vi "connect.vi"(3 "Connect":bool, 7 "LabVIEW Web Service Request":refnum<class "Web Request.lvclass">) -> ()   [LabVIEW 2014]
uses:
  <vilib>/wsapi/Web Request.lvclass
  controls/UI DataSam.ctl
panel:
  # "Use the Web Service Request input terminal to call the VIs on the Web Services palette. Do not remove it from the connector pane unless you don't need access to the palette."
  # "Each additional control wired to the connector pane will be available as an input in the URL. To include an indicator in terminal-mode output (the default setting), it must also be wired to the connector pane."
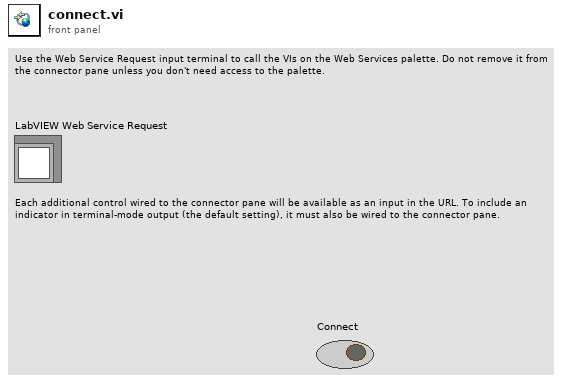
[diagram p1: front panel]
types:
  T1 = typedef "UI DataSam.ctl" = cluster{"Message":string, "Data":variant}
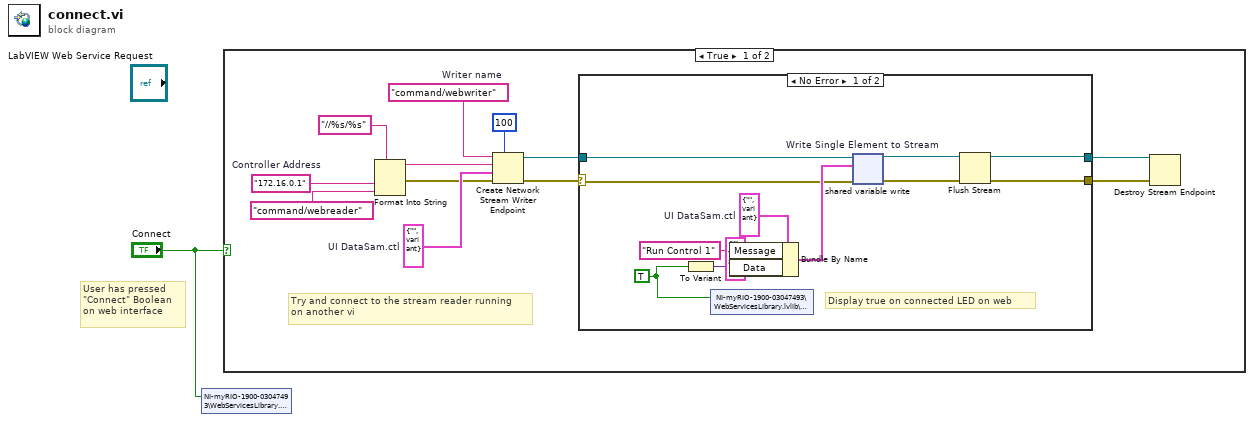
[diagram p0: block diagram]
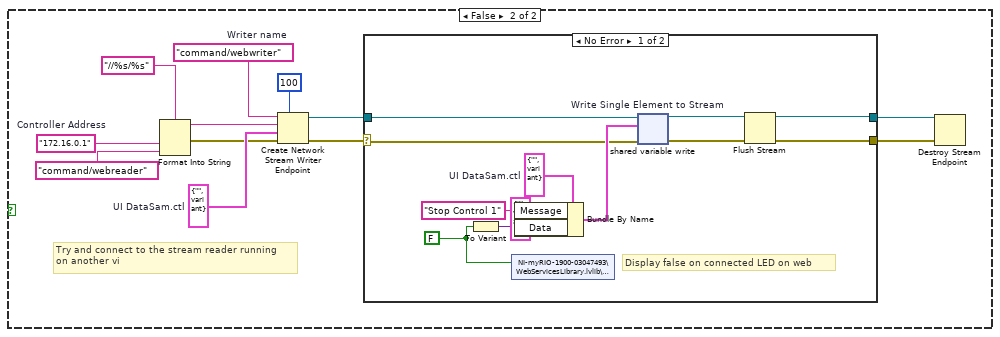
[diagram p3: hidden frame]
diagram:
  # "User has pressed\n\"Connect\" Boolean\non web interface"
  n1 = shared-variable "NI-myRIO-1900-03047493\\WebServicesLibrary.lvlib\\Connect"("Connect") -> ()  [unwired: 1 in, 1 out]
  n2 = case shown="True" "Connect" {
    frame True {
      w13 = "172.16.0.1"  # Controller Address
      w10 = T1 {"Message"="", "Data"=variant}  # UI DataSam.ctl
      w9 = "command/webwriter"  # Writer name
      (unwired) T1 {"Message"="", "Data"=variant} ("UI DataSam.ctl")
      # "Try and connect to the stream reader running\non another vi"
      n3 = Format Into String(format string="//%s/%s", w13, "command/webreader" ("input 2")) -> (resulting string=w7:string, error out=w6:errorcluster)  [unwired: 2 in]
      n4 = Create Network Stream Writer Endpoint(7:100 ("writer buffer size"), 8:w6, 9:w10, 10:w7, 11:w9) -> (0:w12:errorcluster, 3:w11:refnum<k21>)  [unwired: 2 in]
      n5 = case shown="No Error" w12 {
        selector: w12 -> [w15 w25]
        tunnel: w11 -> [w20 w26]
        tunnel: [w19 w26] -> w3
        tunnel: [w18 w25] -> w2
        frame No Error {
          w14 = TRUE
          w17 = T1 {"Message"="", "Data"=variant}  # UI DataSam.ctl
          # "Display true on connected LED on web"
          n6 = To Variant(anything=w14) -> (Variant=w24:variant)
          n7 = shared-variable "NI-myRIO-1900-03047493\\WebServicesLibrary.lvlib\\Connected"(w14) -> ()  [unwired: 1 in, 1 out]
          n8 = Bundle By Name(cluster=w17, "Message"="Run Control 1", "Data"=w24) -> (w16:T1)
          n9 = shared-variable-write "Write Single Element to Stream"(w20, w15, w16) -> (w22:refnum<k21>, w21:errorcluster)  [unwired: 1 in, 1 out]
          n10 = Flush Stream(8:w21, 11:w22) -> (0:w18:errorcluster, 3:w19:refnum<k21>)  [unwired: 2 in, 1 out]
        }
        frame Error {
        }
      }
      n11 = Destroy Stream Endpoint(8:w2, 11:w3) -> ()  [unwired: 1 out]
    }
    frame False {
      w38 = "172.16.0.1"  # Controller Address
      w35 = T1 {"Message"="", "Data"=variant}  # UI DataSam.ctl
      w34 = "command/webwriter"  # Writer name
      (unwired) T1 {"Message"="", "Data"=variant} ("UI DataSam.ctl")
      # "Try and connect to the stream reader running\non another vi"
      n12 = Format Into String(format string="//%s/%s", w38, "command/webreader" ("input 2")) -> (resulting string=w32:string, error out=w31:errorcluster)  [unwired: 2 in]
      n13 = Create Network Stream Writer Endpoint(7:100 ("writer buffer size"), 8:w31, 9:w35, 10:w32, 11:w34) -> (0:w37:errorcluster, 3:w36:refnum<k21>)  [unwired: 2 in]
      n14 = case shown="No Error" w37 {
        selector: w37 -> [w40 w50]
        tunnel: w36 -> [w45 w51]
        tunnel: [w44 w51] -> w28
        tunnel: [w43 w50] -> w27
        frame No Error {
          w39 = FALSE
          w42 = T1 {"Message"="", "Data"=variant}  # UI DataSam.ctl
          # "Display false on connected LED on web"
          n15 = To Variant(anything=w39) -> (Variant=w49:variant)
          n16 = shared-variable "NI-myRIO-1900-03047493\\WebServicesLibrary.lvlib\\Connected"(w39) -> ()  [unwired: 1 in, 1 out]
          n17 = Bundle By Name(cluster=w42, "Message"="Stop Control 1", "Data"=w49) -> (w41:T1)
          n18 = shared-variable-write "Write Single Element to Stream"(w45, w40, w41) -> (w47:refnum<k21>, w46:errorcluster)  [unwired: 1 in, 1 out]
          n19 = Flush Stream(8:w46, 11:w47) -> (0:w43:errorcluster, 3:w44:refnum<k21>)  [unwired: 2 in, 1 out]
        }
        frame Error {
        }
      }
      n20 = Destroy Stream Endpoint(8:w27, 11:w28) -> ()  [unwired: 1 out]
    }
  }
